vi "externalAqcuisitionStart.vi"(8 "error in (no error)":errorcluster) -> (0 "error out":errorcluster, 3 "message out":T1)   [LabVIEW 2017, in "externalAquisition.lvlib"]
uses:
  externalAquisition.lvlib
  programControl/Notifier/TypeDefs/notificationMessage.ctl
  programControl/Notifier/TypeDefs/notifierFGVStates.ctl
  programControl/programControl.lvlib
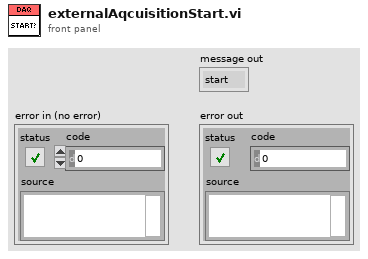
[diagram p1: front panel]
types:
  T1 = typedef "programControl.lvlib/notificationMessage.ctl" = enum16{"start", "wait", "run", "end"}
  T2 = typedef "programControl.lvlib/notifierFGVStates.ctl" = enum16{"obtain", "send", "wait for notification", "release"}
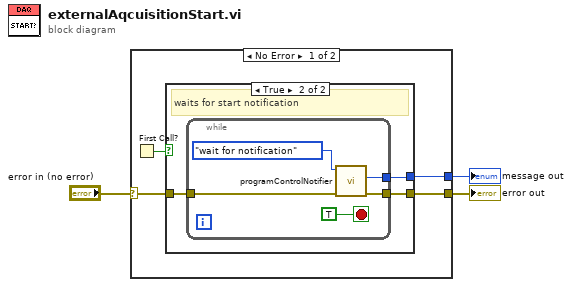
[diagram p0: block diagram]
diagram:
  n1 = case shown="No Error" "error in (no error)" {
    selector: "error in (no error)" -> [w4 w17]
    tunnel: [w7 w17] -> w3
    tunnel: [w6 _] -> w2
    frame No Error {
      n2 = First Call?() -> (First Call?: T/F=w5:bool)
      n3 = case shown="True" w5 {
        tunnel: w4 -> [w8 w11]
        tunnel: [w8 w10] -> w7
        tunnel: [_ w9] -> w6
        frame False {
        }
        frame True {
          # "waits for start notification"
          n4 = while {
            tunnel: w11 -> [w16]
            tunnel: [w13] -> w10
            tunnel: [w12] -> w9
            stop <- TRUE stop-if-true
            n5 = call "programControlNotifier.vi"("error in (no error)"=w16, "Enum"=notifierFGVStates."wait for notification") -> ("error out"=w13:errorcluster, "message out"=w12:T1)  [unwired: 8 in]
          }
        }
      }
    }
    frame Error {
    }
  }
  "error out" <- w3
  "message out" <- w2
